vi "new document.vi"(5 "name":string) -> (4 "Device Out":T1, 6 "id":string, 15 "error out":errorcluster)   [LabVIEW 2019]
uses:
  <userlib>/IoT Devices/_subVIs/HTTPComm.ctl
  <userlib>/Onshape/_SubVI/Cluster.ctl
panel:
  in  "Device In":T1
  out "Comm":T2
  in  "error in":errorcluster
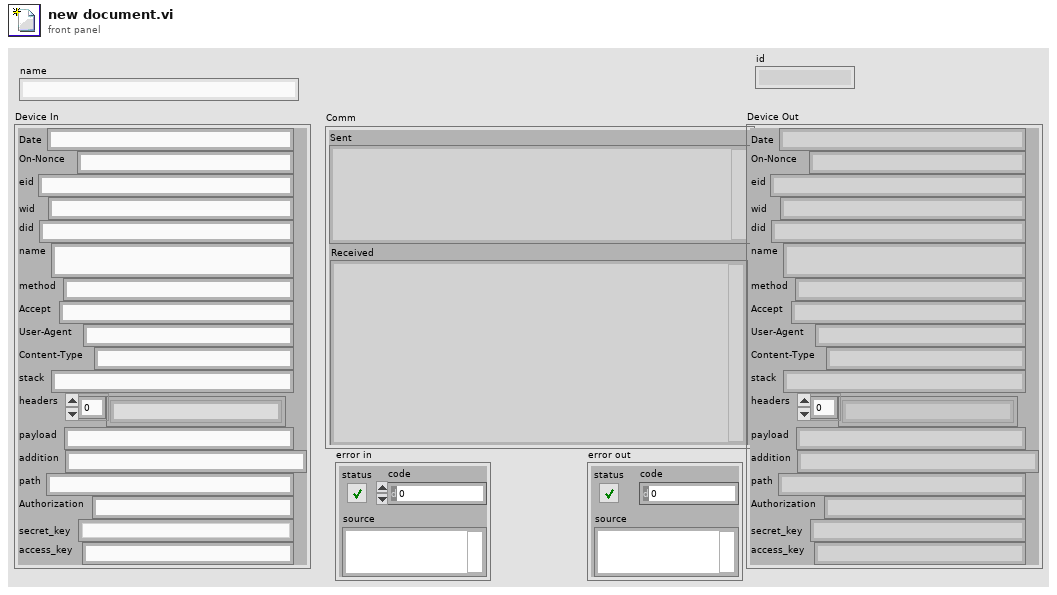
[diagram p1: front panel]
types:
  T1 = typedef "Cluster.ctl" = cluster{"Date":string, "On-Nonce":string, "eid":string, "wid":string, "did":string, "name":string, "method":string, "Accept":string, "User-Agent":string, "Content-Type":string, "stack":string, "headers":string[], "payload":string, "addition":string, "path":string, "Authorization":string, "secret_key":string, "access_key":string}
  T2 = typedef "HTTPComm.ctl" = cluster{"url":string, "sent headers":string, "sent body":string, "headers":string, "body":string, "Sent":string, "Received":string}
  T3 = cluster{"name":string, "defaultWorkspace":cluster{"documentId":string, "id":string}}
  T4 = cluster{"name":string, "ownerType":i32, "isPublic":bool}
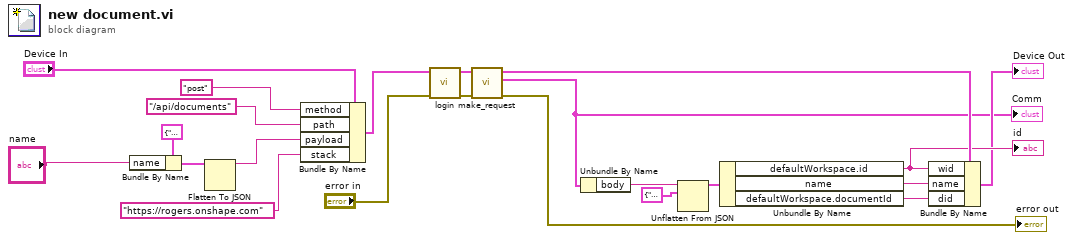
[diagram p0: block diagram]
diagram:
  n1 = Bundle By Name(cluster=T4 {"name"="", "ownerType"=0, "isPublic"=FALSE}, "name"="name") -> (w22:T4)
  n2 = Flatten To JSON(anything=w22) -> (JSON string=w18:string)  [unwired: 2 in, 1 out]
  n3 = Bundle By Name(cluster="Device In", "method"="post" ("Method"), "path"="/api/documents" ("payload"), "payload"=w18, "stack"="https://rogers.onshape.com" ("stacks")) -> (w12:T1)
  n4 = call <userlib>:"login.vi"("error in"="error in", "Device In"=w12) -> ("error out"=w10:errorcluster, "Device Out"=w11:T1)  [unwired: 8 in]
  n5 = call <userlib>:"make_request.vi"("Error in"=w10, "Device In"=w11) -> ("error out"=→"error out":errorcluster, "Comm"=w3:T2, "Device Out"=w13:T1)  [unwired: 6 in, 1 out]
  "Comm" <- w3
  n6 = Unbundle By Name(w3) -> ("body"=w15:string)
  n7 = Unflatten From JSON(JSON string=w15, type and defaults=T3 {"name"="", "defaultWorkspace"={"documentId"="", "id"=""}}) -> (value=w14:T3)  [unwired: 5 in, 1 out]
  n8 = Unbundle By Name(w14) -> ("defaultWorkspace.id"=w7:string, "name"=w9:string, "defaultWorkspace.documentId"=w8:string)
  "id" <- w7
  n9 = Bundle By Name(cluster=w13, "wid"=w7, "name"=w9, "did"=w8) -> (→"Device Out":T1)
